vi "ad analog out.vi"(7 "data":sgl, 8 "error in (no error)":errorcluster, 9 "range":i32, 10 "cha":i32, 11 "adh":i32) -> (0 "error out":errorcluster, 3 "function return":i32)   [LabVIEW 2021, in "libad4.lvlib"]
doc: "LLIBAD4 function: ad_analog_out (int32_t adh, int32_t cha, int32_t range, float data);\n\nThis function converts the voltage value with ad_float_to_sample() and then calls ad_discrete_out(). Only analog outputs are supported, i.e. AD_CHA_TYPE_ANALOG_OUTIN|cha is internally used as channel number."
uses:
  <userlib>/libad4/libad4.lvlib
  <userlib>/libad4/libad4.dll
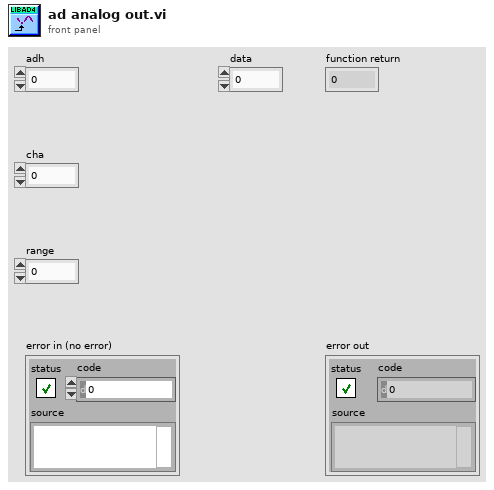
[diagram p1: front panel]
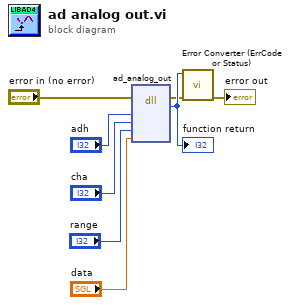
[diagram p0: block diagram]
diagram:
  n1 = dll-call lib="C:/Program Files/National Instruments/LabVIEW 2021/user.lib/libad4/libad4.*" fn="ad_analog_out"(error in="error in (no error)", "adh"="adh", "cha"="cha", "range"="range", "data"="data") -> (error out=w2:errorcluster, w8:i32)  [unwired: 6 in, 1 out]
  "function return" <- w8
  n2 = call <userlib>:"Error Converter (ErrCode or Status).vi"("error in (no error)"=w2, "error code"=w8) -> ("error out"=→"error out":errorcluster)  [unwired: 9 in]
